vi "New Report Page.vi"(0 "report in":refnum<class "NI_HTML.lvclass">, 9 "MS Office parameters":T1, 11 "error in (no error)":errorcluster) -> (4 "report out":refnum<class "NI_HTML.lvclass">, 15 "error out":errorcluster)   [LabVIEW 2017, in "NI_HTML.lvclass"]
doc: "Creates a page break within the report."
uses:
  <vilib>/Utility/NIReport.llb/HTML/NI_HTML.lvclass
  <vilib>/Utility/NIReport.llb/HTML/NI_HTML.lvclass/NI_HTML.ctl
  <vilib>/Utility/NIReport.llb/NI_ReportGenerationCore.lvlib
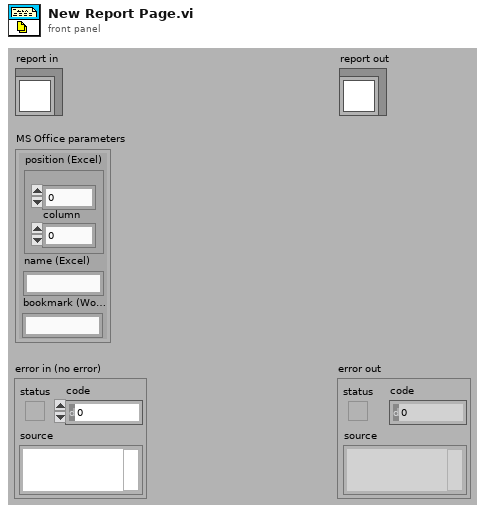
[diagram p1: front panel]
types:
  T1 = cluster{"position (Excel)":cluster{"row":i32, "column":i32}, "name (Excel) ":string, "bookmark (Word)":string}
  T2 = typedef "NI_ReportGenerationCore.lvlib/HTML Report Data.ctl" = cluster{"Body Text":string, "Font Tag":string, "Title Text":string, "Header Text":string, "Footer Text":string, "Image List":path[]}
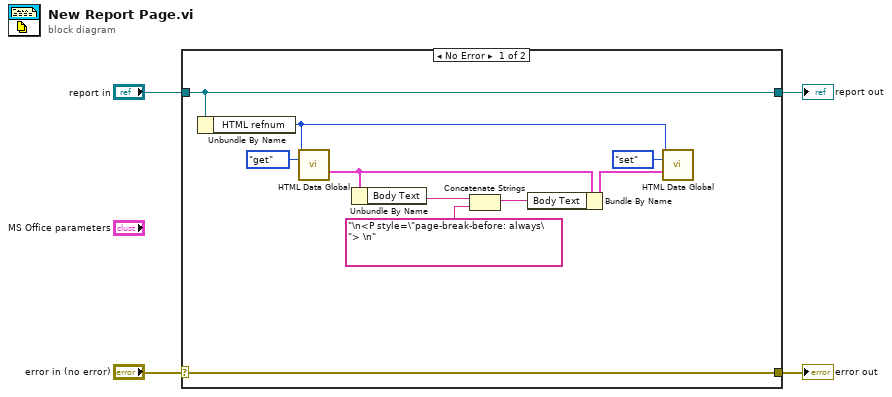
[diagram p0: block diagram]
diagram:
  n1 = case shown="No Error" "error in (no error)" {
    selector: "error in (no error)" -> [w14 w16]
    tunnel: [w14 w16] -> w3
    tunnel: [w9 w15] -> w1
    tunnel: "report in" -> [w9 w15]
    frame No Error {
      n2 = Unbundle By Name(w9) -> ("HTML refnum"=w5:u32)
      n3 = call <vilib>:"HTML Data Global.vi"("HTML refnum"=w5, "menu"=enum16{"init", "get", "set", "delete"}."get") -> ("HTML report data out"=w7:T2)  [unwired: 1 in, 12 out]
      n4 = Unbundle By Name(w7) -> ("Body Text"=w13:string)
      n5 = Concatenate Strings(w13, "\n<P style=\"page-break-before: always\"> \n") -> (w12:string)
      n6 = Bundle By Name(cluster=w7, "Body Text"=w12) -> (w6:T2)
      n7 = call <vilib>:"HTML Data Global.vi"("HTML refnum"=w5, "menu"=enum16{"init", "get", "set", "delete"}."set", "HTML report data in"=w6) -> ()  [unwired: 13 out]
    }
    frame Error {
    }
  }
  "error out" <- w3
  "report out" <- w1
